vi "addition.vi"() -> ()   [LabVIEW 2012]
panel:
  in  "Tab Control":T1(tab)
  in  "Numeric 2":dbl
  in  "Numeric":dbl
  out "x+y":dbl
  out "Waveform Graph":dynamicdata(graph)
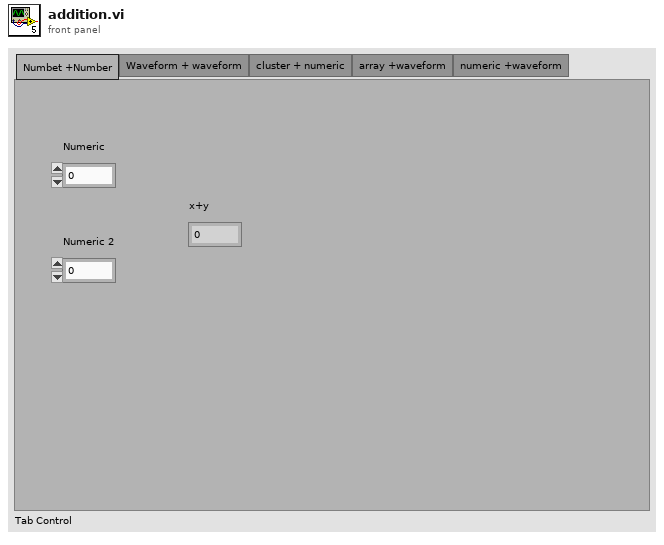
[diagram p1: front panel]
types:
  T1 = enum32{"Numbet +Number", "Waveform + waveform", "cluster + numeric", "array +waveform", "numeric +waveform"}
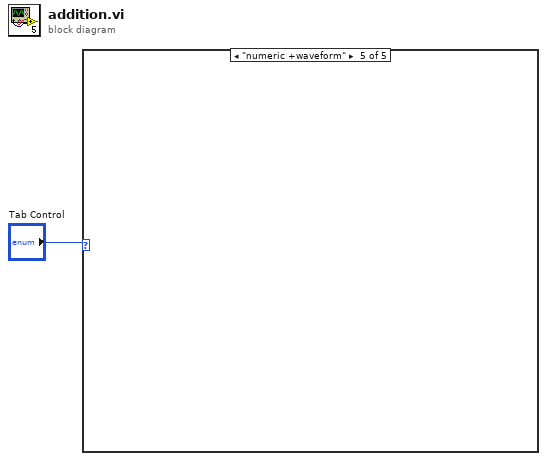
[diagram p0: block diagram]
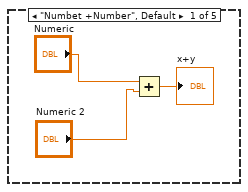
[diagram p2: hidden frame]
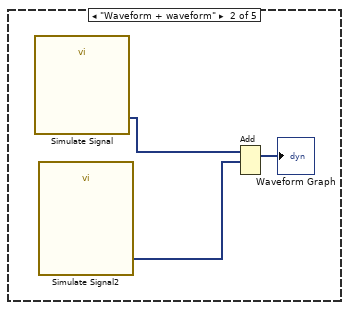
[diagram p3: hidden frame]
diagram:
  n1 = case shown="\"numeric +waveform\"" "Tab Control" {
    frame "Numbet +Number", Default {
      n2 = Add(x="Numeric", y="Numeric 2") -> (x+y=→"x+y":dbl)
    }
    frame "Waveform + waveform" {
      n3 = call "Simulate Signal"() -> ("Sine"=w7:dynamicdata)  [unwired: 14 in, 1 out]
      n4 = call "Simulate Signal2"() -> ("Sine"=w6:dynamicdata)  [unwired: 14 in, 1 out]
      n5 = Add(1:w6, 2:w7) -> (0:→"Waveform Graph":dynamicdata)  [unwired: 1 in, 1 out]
    }
    frame "cluster + numeric" {
    }
    frame "array +waveform" {
    }
    frame "numeric +waveform" {
    }
  }
